vi "VD_Init.vi"(8 "error in":errorcluster) -> (0 "error out":errorcluster, 3 "VISA Vd_Supply":refnum<visa-resource-name>)   [LabVIEW 2017]
uses:
  Agilent E364X Series.lvlib
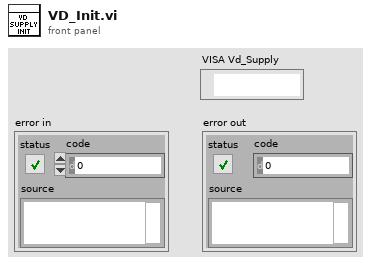
[diagram p1: front panel]
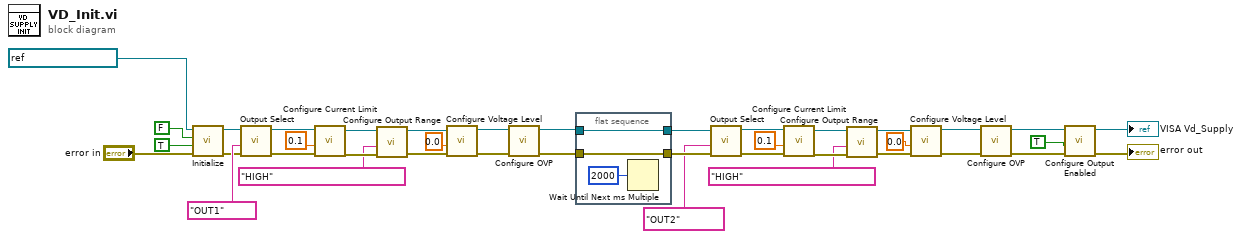
[diagram p0: block diagram]
diagram:
  n1 = call "Initialize.vi"("error in (no error)"="error in", "ID Query (T: Query)"=TRUE, "Reset Device (T: Reset)"=FALSE, "VISA resource name"=refnum<visa-resource-name> "GPIB0::5::INSTR" ("Instrument Resource Name")) -> ("error out"=w17:errorcluster, "VISA resource name out"=w12:refnum<visa-resource-name>)  [unwired: 6 in]
  n2 = call "Output Select.vi"("error in (no error)"=w17, "Instrument Select (Output 1)"="OUT1", "VISA resource name"=w12) -> ("error out"=w20:errorcluster, "VISA resource name out"=w19:refnum<visa-resource-name>)  [unwired: 7 in]
  n3 = call "Configure Current Limit.vi"("error in (no error)"=w20, "Current Limit (0.0 Amps)"=0.1, "VISA resource name"=w19) -> ("error out"=w35:errorcluster, "VISA resource name out"=w34:refnum<visa-resource-name>)  [unwired: 7 in]
  n4 = call "Configure Output Range.vi"("error in (no error)"=w35, "Range (High Voltage / Low Current)"="HIGH", "VISA resource name"=w34) -> ("error out"=w28:errorcluster, "VISA resource name out"=w27:refnum<visa-resource-name>)  [unwired: 7 in]
  n5 = call "Configure Voltage Level.vi"("error in (no error)"=w28, "Level (0.0 Volts)"=0.0, "VISA resource name"=w27) -> ("error out"=w5:errorcluster, "VISA resource name out"=w8:refnum<visa-resource-name>)  [unwired: 7 in]
  n6 = call "Configure OVP.vi"("error in (no error)"=w5, "VISA resource name"=w8) -> ("error out"=w6:errorcluster, "VISA resource name out"=w7:refnum<visa-resource-name>)  [unwired: 8 in]
  n7 = flat-sequence {
    tunnel: [w41] -> w15
    tunnel: w6 -> [w41]
    tunnel: [w40] -> w9
    tunnel: w7 -> [w40]
    frame #0 {
      n8 = Wait Until Next ms Multiple(millisecond multiple=u32 2000) -> ()  [unwired: 1 out]
    }
  }
  n9 = call "Output Select.vi"("error in (no error)"=w15, "Instrument Select (Output 1)"="OUT2", "VISA resource name"=w9) -> ("error out"=w16:errorcluster, "VISA resource name out"=w14:refnum<visa-resource-name>)  [unwired: 7 in]
  n10 = call "Configure Current Limit.vi"("error in (no error)"=w16, "Current Limit (0.0 Amps)"=0.1, "VISA resource name"=w14) -> ("error out"=w31:errorcluster, "VISA resource name out"=w30:refnum<visa-resource-name>)  [unwired: 7 in]
  n11 = call "Configure Output Range.vi"("error in (no error)"=w31, "Range (High Voltage / Low Current)"="HIGH", "VISA resource name"=w30) -> ("error out"=w23:errorcluster, "VISA resource name out"=w24:refnum<visa-resource-name>)  [unwired: 7 in]
  n12 = call "Configure Voltage Level.vi"("error in (no error)"=w23, "Level (0.0 Volts)"=0.0, "VISA resource name"=w24) -> ("error out"=w4:errorcluster, "VISA resource name out"=w2:refnum<visa-resource-name>)  [unwired: 7 in]
  n13 = call "Configure OVP.vi"("error in (no error)"=w4, "VISA resource name"=w2) -> ("error out"=w3:errorcluster, "VISA resource name out"=w1:refnum<visa-resource-name>)  [unwired: 8 in]
  n14 = call "Configure Output Enabled.vi"("error in (no error)"=w3, "Output Enabled (F: Off)"=TRUE, "VISA resource name"=w1) -> ("error out"=→"error out":errorcluster, "VISA resource name out"=→"VISA Vd_Supply":refnum<visa-resource-name>)  [unwired: 7 in]
